vi "SplashWnd - Module Starting Up.vi"(7 "Title":string, 8 "Error In (No Error)":errorcluster, 9 "Name (\"\" to Use UUID)":string="SplashWindow", 11 "Modules":string[](array[string])) -> (0 "error out":errorcluster)   [LabVIEW 2020, in "CSM-SplashWindow.lvlib"]
uses:
  79d02799-5e27-450a-8f22-22593f2d7556.vi
  SplashWindow.vi
  <userlib>/_NEVSTOP/Communicable State Machine(CSM)/addons/API-String-Arugments-Support/_Support/Data To API String Arguments.vi
  CSM-SplashWindow.lvlib
  <userlib>/_NEVSTOP/Communicable State Machine(CSM)/Communicable State Machine.lvlib
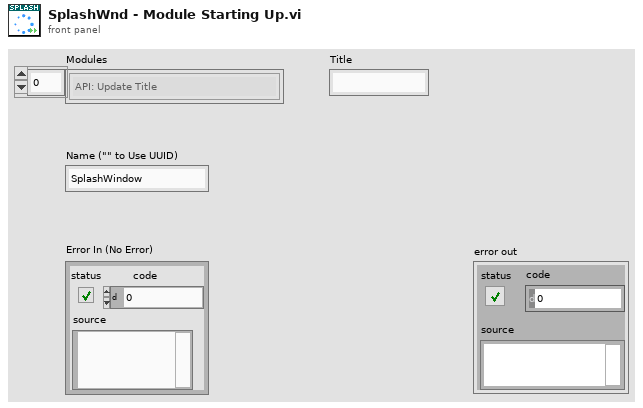
[diagram p1: front panel]
types:
  T1 = enum32{"Invalid", "Default", "Floating", "Floating/Auto-Hide", "Modal"}
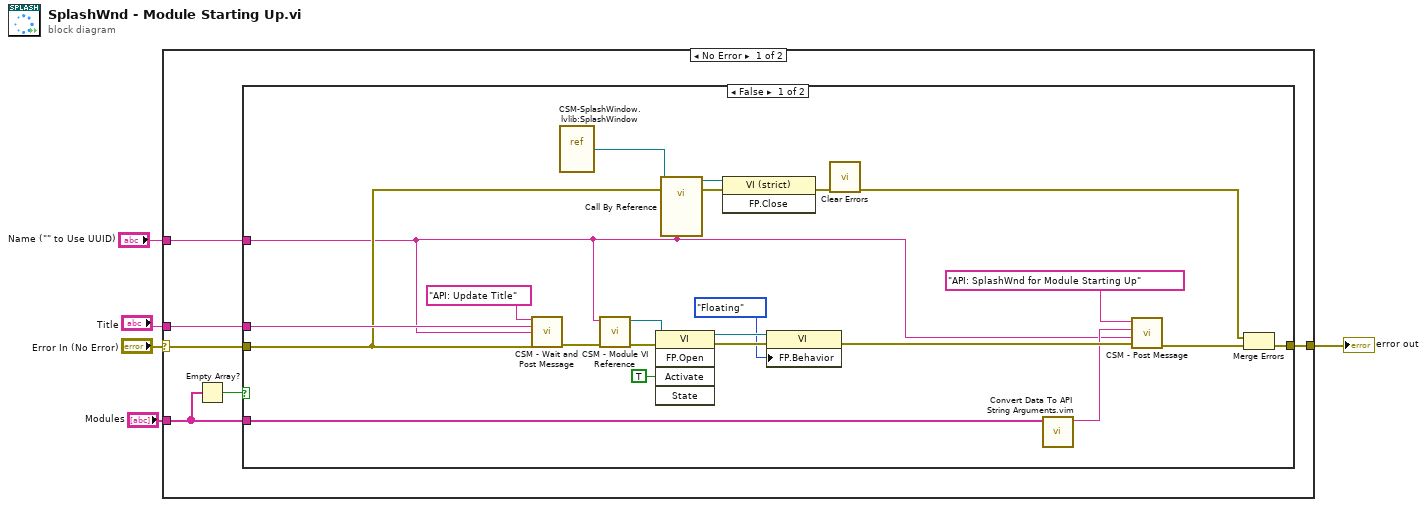
[diagram p0: block diagram]
diagram:
  n1 = case shown="No Error" "Error In (No Error)" {
    selector: "Error In (No Error)" -> [w10 w35]
    tunnel: "Title" -> [w11 _]
    tunnel: [w9 w35] -> w3
    tunnel: "Modules" -> [w8 _]
    tunnel: "Name (\"\" to Use UUID)" -> [w6 _]
    frame No Error {
      n2 = Empty Array?(array=w8) -> (empty?=w7:bool)
      n3 = case shown="False" w7 {
        tunnel: w11 -> [w32 _]
        tunnel: w10 -> [w24 w34]
        tunnel: [w20 w34] -> w9
        tunnel: w8 -> [w17 _]
        tunnel: w6 -> [w12 _]
        frame False {
          n4 = call <userlib>:"CSM - Wait and Post Message.vi"("State"="API: Update Title", "Arguments (\"\")"=w32, "Target Module"=w12, "Error In (No Error)"=w24) -> ("error out"=w31:errorcluster)  [unwired: 10 in, 1 out]
          n5 = vi-ref "CSM-SplashWindow.lvlib:SplashWindow.vi"() -> (w25:refnum<vi>)
          n6 = call <userlib>:"CSM - Module VI Reference.vi"("error in (no error)"=w31, "CSM Name"=w12) -> ("error out"=w29:errorcluster, "CSM Module VIRef"=w30:refnum<vi>)  [unwired: 8 in]
          n7 = invoke class="VI" method="FP.Open"(reference=w30, error in=w29, "Activate"=TRUE ("Activate?")) -> (reference out=w27:refnum<vi>, error out=w28:errorcluster)  [unwired: 2 in, 3 out]
          n8 = call-by-ref "?"(reference=w25, error in=w24, "Name (\"\" to Use UUID)"=w12) -> (reference out=w14:refnum<vi>, error out=w19:errorcluster)  [unwired: 11 in]
          n9 = invoke class="VI (strict)" method="FP.Close"(reference=w14, error in=w19) -> (error out=w15:errorcluster)  [unwired: 1 in, 2 out]
          n10 = property class="VI"(reference=w27, error in=w28, "FP.Behavior"=T1."Floating" ("Front Panel Window:Behavior")) -> (error out=w23:errorcluster)  [unwired: 1 out]
          n11 = call <vilib>:"Clear Errors.vi"("error in (no error)"=w15) -> ("error out"=w13:errorcluster)  [unwired: 5 in, 1 out]
          n12 = call "Convert Data To API String Arguments.vim"("Data"=w17) -> ("API String"=w18:string)  [unwired: 7 in, 1 out]
          n13 = call <userlib>:"CSM - Post Message.vi"("Error In (No Error)"=w23, "Target Module"=w12, "Arguments (\"\")"=w18, "State"="API: SplashWnd for Module Starting Up") -> ("error out"=w21:errorcluster)  [unwired: 7 in]
          n14 = Merge Errors(w13, w21) -> (w20:errorcluster)
        }
        frame True {
        }
      }
    }
    frame Error {
    }
  }
  "error out" <- w3
